vi "trace_header.vi"() -> (2 "Header":sgl[](array[numeric]))   [LabVIEW 2013]
uses:
  probe_point.ctl
  initialization/micron_globals.vi
panel:
  # "Trace magic 123.125 (fixed)"
  # "Trace data version.  1.3, or whatever."
  # "Size of data records to follow, in vectors of three single-floats (12 bytes).  \nAdd 1 to include this header."
  # "Return what the trace data header should be.  This is put at the beginning of a trace file and on each packet sent out over the net."
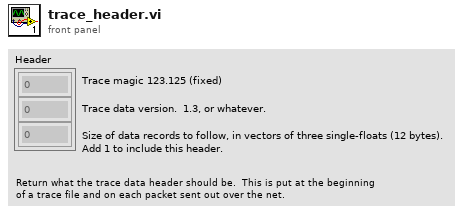
[diagram p1: front panel]
types:
  T1 = typedef "probe_point.ctl" = enum16{"Position (tip)", "Position (RCM)", "Null pos (tip)", "Null pos (RCM)", "V limiter (tip)", "V Limiter (RCM)", "Goal (tip)", "Goal (RCM)", "Link pos 0", "Link pos 1", "KF link pos 0", "KF link pos 1", "Link rate 0", "Link rate 1", "Link residue 0", "Link residue 1", "Link goal 0", "Link goal 1", "Rate limit 0", "Rate limit 1", "Link error 0", "Link error 1", "Controller 0", "Controller 1", "Output 0", "Output 1", "Drive 0", "Drive 1", "Stimulus 0", "Stimulus 1", "Trace data 0", "Trace data 1", "Analog data 0", "Analog data 1", "Status flags", "Light 0", "Light 1", "Light 2", "Light 3", "Light 4", "Light 5", "Goal origin", "Goal rotation 0", "Goal rotation 1", "Goal rotation 2", "Output origin", "Output rotation 0", "Output rotation 1", "Output rotation 2", "Handle origin", "Handle rotation 0", "Handle rotation 1", "Handle rotation 2", "Handle position", "Handle velocity", "Handle acceleration", "Handle angles", "Handle angle rates", "Handle pos residue", "Handle angle residue", "Trace length"}
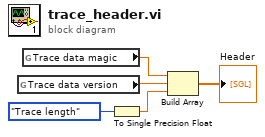
[diagram p0: block diagram]
diagram:
  n1 = global read "micron_globals.vi" "Trace data version"() -> (w4:sgl)
  n2 = global read "micron_globals.vi" "Trace data magic"() -> (w3:sgl)
  n3 = To Single Precision Float(number=probe_point."Trace length" ("Probe point")) -> (single precision float=w1:sgl)
  n4 = Build Array(w3, w4, w1) -> (→"Header":sgl[])
